vi "ECG Zoom Window.vi"(8 "error in (no error)":errorcluster, 9 "ECG Waveform Data":dbl[](array[numeric])=array[5000 elements], 10 "Plot Color":u32, 11 "ECG Signal IN":string) -> (0 "error out":errorcluster)   [LabVIEW 2010]
doc: "This VI serves as a pop-up window to display a single ECG signal with the data shown as is (not normalized).\n\nInputs:\nECG Signal IN - (str) name of signal being displayed\nPlot Color - (I32) value of color to display plot as\nECG Waveform Data - (DBL[]) data for ECG plot\nerror in - error input cluster\n\nOutput:\nerror out - error output cluster"
panel:
  in  "Exit":bool
  out "ECG Signal":string
  out "ECG Waveform":dbl[](graph)
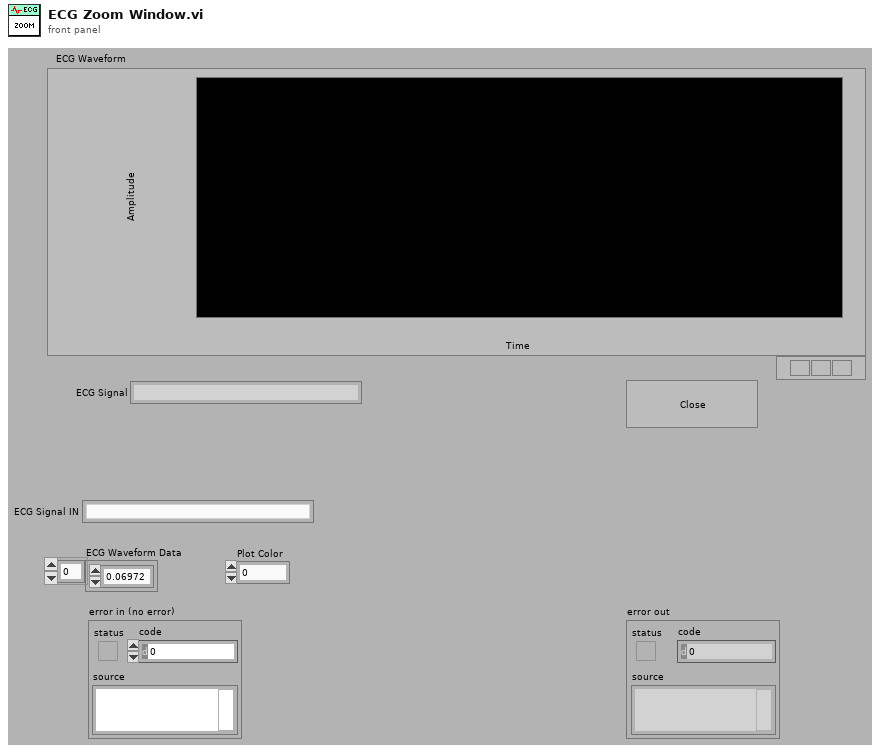
[diagram p1: front panel]
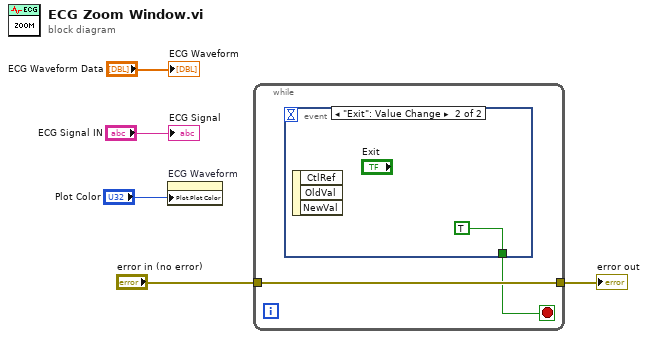
[diagram p0: block diagram]
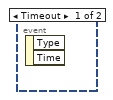
[diagram p2: hidden frame]
diagram:
  n1 = property on="ECG Waveform" class="WFGraph (strict)"("Plot.Plot Color"="Plot Color") -> ()  [unwired: 2 in, 2 out]
  n2 = while {
    tunnel: "error in (no error)" -> [w7]
    tunnel: [w7] -> w2
    stop <- w6 stop-if-true
    n3 = event shown="[1] \"Exit\": Value Change" {
      selector: _ -> [_ _]
      dyn-events: _ -> [_ _]
      timeout: _ -> [_ _]
      tunnel: [_ TRUE] -> w6
      event Timeout {
        n4 = event-data() -> ()  [unwired: 3 out]
      }
      event "Exit": Value Change {
        n5 = event-data() -> ()  [unwired: 4 out]
      }
    }
  }
  "error out" <- w2
  "ECG Waveform" <- "ECG Waveform Data"
  "ECG Signal" <- "ECG Signal IN"
